vi "Utest2.vi"() -> ()   [LabVIEW 2010]
panel:
  in  "Boolean":bool=TRUE caption="открывашка"
  out "ViStatusOut":T1
  in  "stop":bool
  out "Waveform Graph":T2(graph)
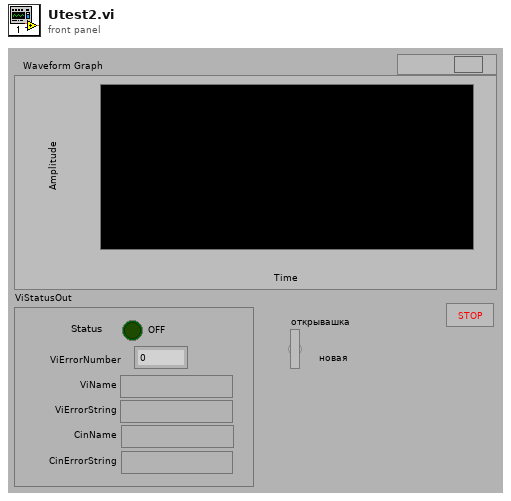
[diagram p1: front panel]
types:
  T1 = cluster{"Status":bool, "ViErrorNumber":u32, "ViName":string, "ViErrorString":string, "CinName":string, "CinErrorString":string}
  T2 = cluster{"dimension size":dbl, "dimension size":dbl, "Buffer":i16[][]}
  T3 = cluster{"DllVersion":u32, "InterfaceType":u32, "InterfaceInstance":u32, "ModuleHandle":u32, "ReadBuffersParsArray":cluster{"Buffer":i16[], "ReadOv":u32, "ReadEvent":u32}[], "WriteBuffersParsArray":cluster{"Buffer":i16[], "WriteOv":u32, "WriteEvent":u32}[]}
  T4 = cluster{"Buffer":i16[], "ReadOv":u32, "ReadEvent":u32}[]
  T5 = cluster{"Buffer":i16[], "ReadOv":u32, "ReadEvent":u32}
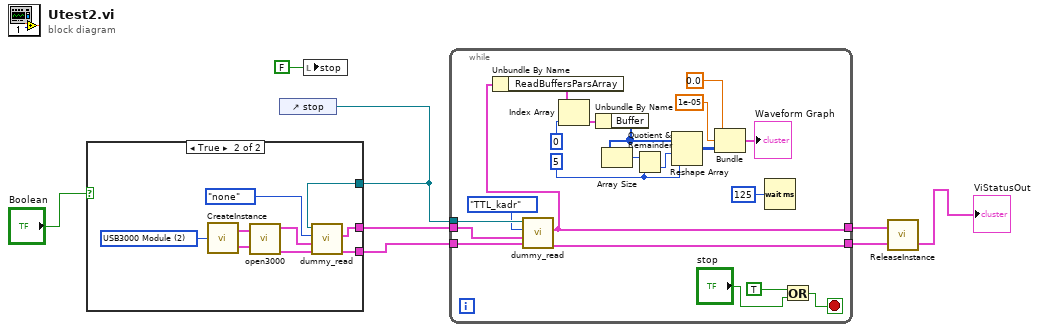
[diagram p0: block diagram]
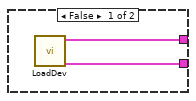
[diagram p2: hidden frame]
diagram:
  n1 = control-ref of="stop"() -> (w1:refnum<vi>)
  n2 = case shown="True" "Boolean" {
    tunnel: [w9 w14] -> w5
    tunnel: [w10 w13] -> w4
    tunnel: w1 -> [_ w12]
    frame False {
      n3 = call "LoadDev.vi"() -> ("ViStatus"=w9:T1, "InterfaceInfo"=w10:T3)  [unwired: 5 in, 1 out]
    }
    frame True {
      w18 = u32 2 items=["Unknown Module", "USB2185 Module", "USB3000 Module"] ("InterfaceType")
      n4 = call "CreateInstance.vi"("InterfaceType"=w18) -> ("InterfaceInfo"=w17:T3, "ViStatus"=w19:T1)
      n5 = call "open3000.vi"("ViInfo"=w19, "InterfaceInfo"=w17) -> ("ViInfoOut"=w15:T1, "InterfaceInfoOut"=w16:T3)  [unwired: 3 in, 1 out]
      n6 = call "dummy_read.vi"("ViStatusOut 2"=w15, "InterfaceInfoOut 2"=w16, "SyncType3000"=enum16{"none", "TTL", "TTL_kadr", "analog"}."none", "Ctrl Reference"=w12) -> ("ViStatusOut"=w14:T1, "InterfaceInfoOut"=w13:T3)  [unwired: 2 in]
    }
  }
  n7 = local write "stop"(FALSE ("stop")) -> ()
  n8 = while {
    tunnel: w1 -> [w26]
    tunnel: w5 -> [w28]
    tunnel: [w24] -> w8
    tunnel: w4 -> [w29]
    tunnel: [w27] -> w7
    stop <- w21 stop-if-true
    w35 = 5 ("dimension size")
    n9 = call "dummy_read.vi"("ViStatusOut 2"=w28, "InterfaceInfoOut 2"=w29, "SyncType3000"=enum16{"none", "TTL", "TTL_kadr", "analog"}."TTL_kadr", "Ctrl Reference"=w26) -> ("ViStatusOut"=w24:T1, "InterfaceInfoOut"=w27:T3)  [unwired: 2 in]
    n10 = Unbundle By Name(w27) -> ("ReadBuffersParsArray"=w40:T4)
    n11 = Index Array(array=w40, index=0) -> (element=w39:T5)
    n12 = Unbundle By Name(w39) -> ("Buffer"=w37:i16[])
    n13 = Array Size(array=w37) -> (size(s)=w36:i32)
    n14 = Quotient & Remainder(x=w36, y=w35) -> (floor(x/y)=w34:i32)  [unwired: 1 out]
    n15 = Reshape Array(w37, w34, w35) -> (w33:i16[][])
    n16 = Bundle("dimension size"=0.0, "dimension size"=1e-05, "Buffer"=w33) -> (→"Waveform Graph":T2)  [unwired: 1 in]
    n17 = Wait (ms)(milliseconds to wait=u32 125) -> ()  [unwired: 1 out]
    n18 = Or(x=TRUE, y="stop") -> (x .or. y?=w21:bool)
  }
  n19 = call "ReleaseInstance.vi"("ViStatusIn"=w8, "InterfaceInfoIn"=w7) -> ("ViStatusOut"=→"ViStatusOut":T1)  [unwired: 1 out]
